vi "Main.vi"() -> ()   [LabVIEW 2013, in "Project Wizard.lvlib"]
doc: "This template is for the Queued Message Handler design pattern.\n\nThe Event Handling Loop generates messages based on user interface actions.\n\nThe Message Handling Loop processes messages generated by the Event Handling Loop, or by other messages. The messages are string values, so new messages can be added easily to the Message Cases case structure in the Message Handling Loop. Each message cluster can also provide an optional value for Message Data, which is a variant that can be converted to whatever message-specific data is required."
uses:
  Project Wizard.lvlib
  controls/UI Data.ctl
  controls/Template.ctl
  support/Message Queue/Enqueue Message (Single).vi
  support/Message Queue/Enqueue Message (Array).vi
  <vilib>/Platform/browser.llb/Open URL in Default Browser (path).vi
  <vilib>/Utility/error.llb/Error Cluster From Error Code.vi
  <vilib>/regexp/Match Regular Expression.xnode
  <vilib>/ErrorRing/Error Ring.xnode
  support/Message Queue/Message Queue.lvlib
  support/User Event - Stop/User Event - Stop.lvlib
panel:
  in  "Tab Control":enum32{"Project", "Properties"}(tab)
  in  "Target IP address or DNS name":string
  in  "Project name":string
  in  "Template":u16(ring) items=["Base", "Base - XNET"]
  in  "Project root folder":path
  in  "ProjFolder":bool
  out "Project path":path
  in  "OpenProj":bool
  in  "Description":string
  in  "Creator":string
  in  "Cancel":bool
  in  "Create":bool
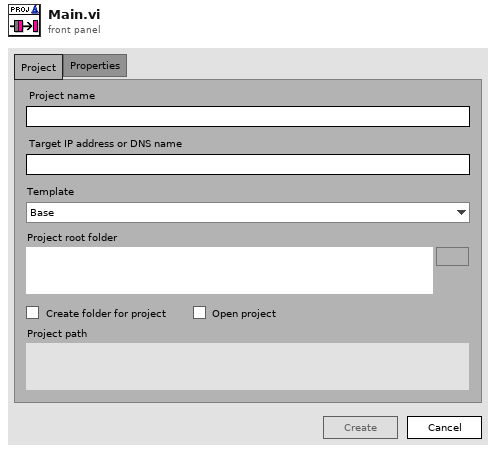
[diagram p1: front panel]
types:
  T1 = typedef "Project Wizard.lvlib/UI Data.ctl" = cluster{"ProjRootFolder":path, "ProjName":string, "Open":bool, "CreateFolder":bool, "Description":string, "Creator":string, "ProjPath":path, "Templates":T2[], "TemplateIdx":u16, "IP":string}
  T2 = typedef "Project Wizard.lvlib/Template.ctl" = cluster{"DispName":string, "Path":path, "DiskName":string}
  T3 = typedef "Project Wizard.lvlib/Message Queue.lvlib/All Message Queues.ctl" = cluster{"UI":refnum<queue>}
  T4 = enum8{"Enabled", "Disabled", "Disabled and Grayed Out"}
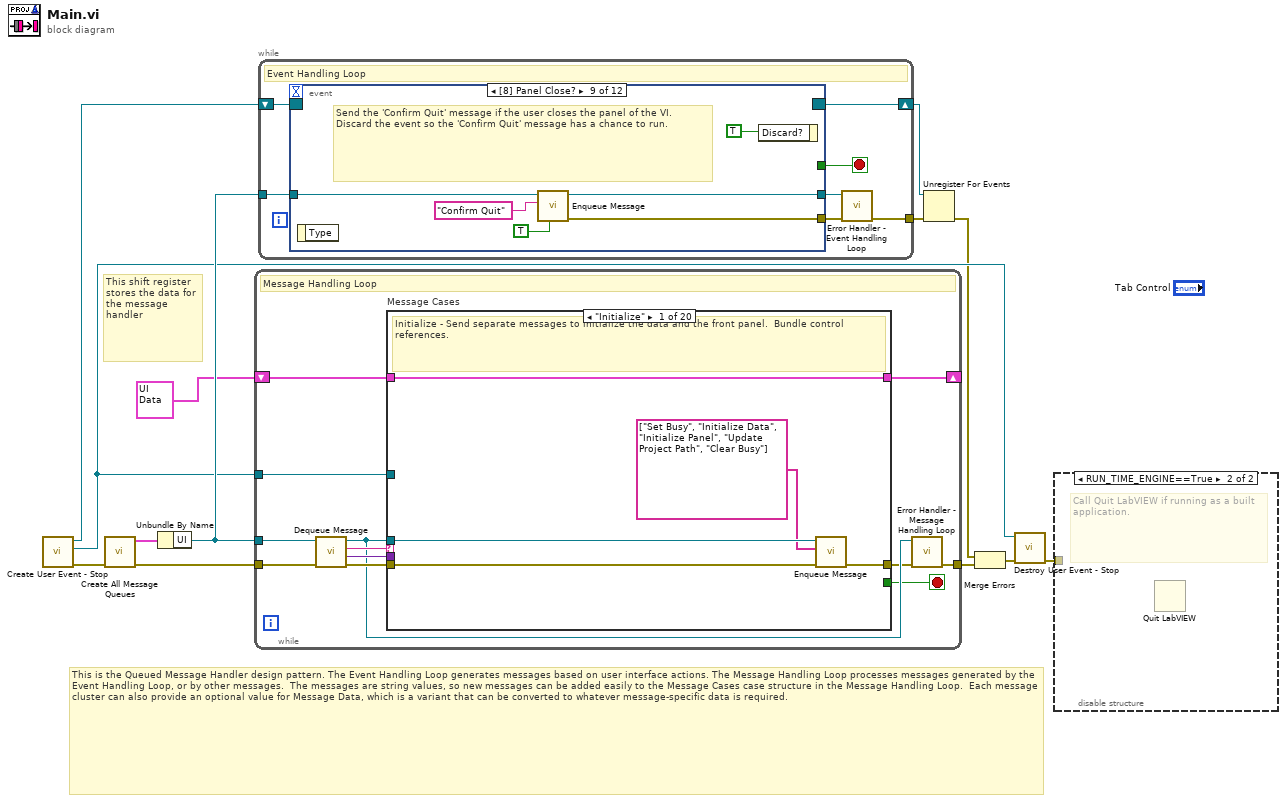
[diagram p0: block diagram]
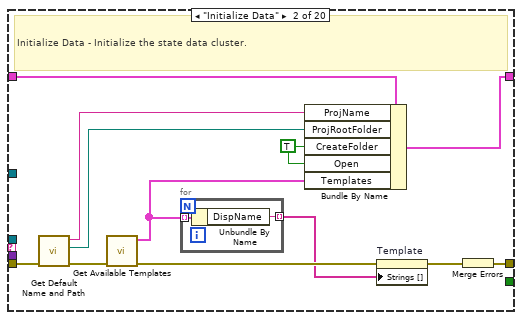
[diagram p2: hidden frame]
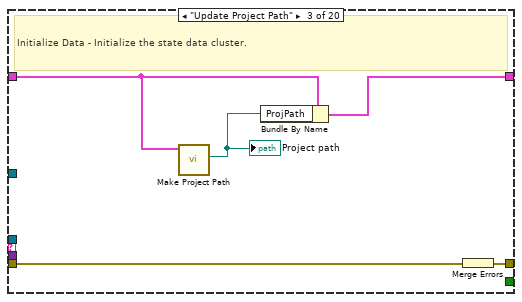
[diagram p3: hidden frame]
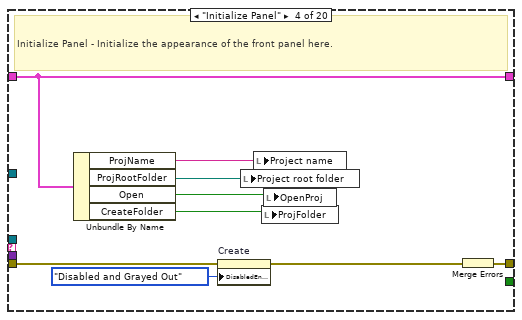
[diagram p4: hidden frame]
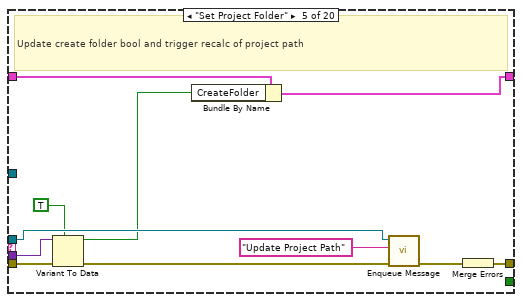
[diagram p5: hidden frame]
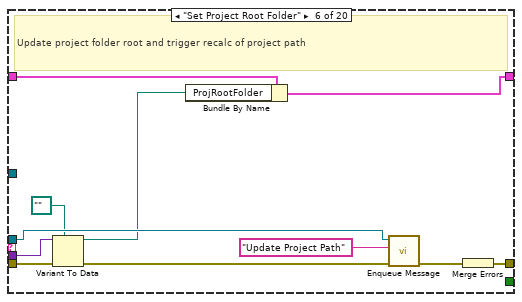
[diagram p6: hidden frame]
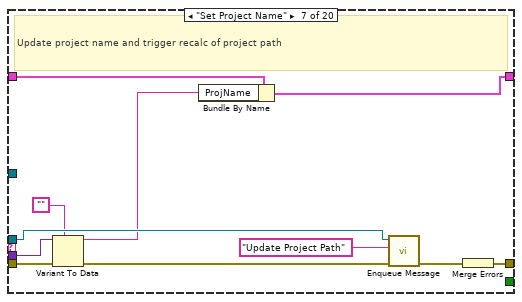
[diagram p7: hidden frame]
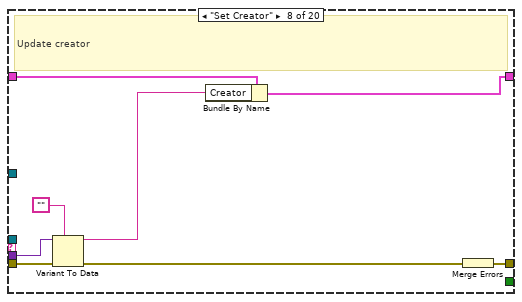
[diagram p8: hidden frame]
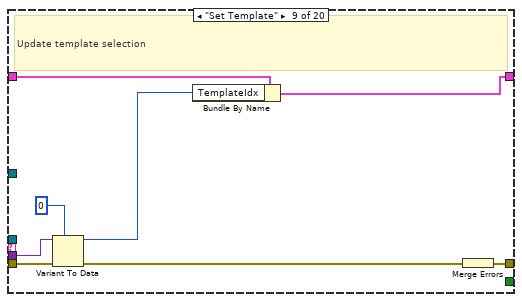
[diagram p9: hidden frame]
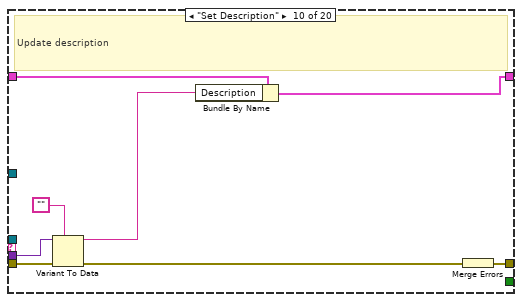
[diagram p10: hidden frame]
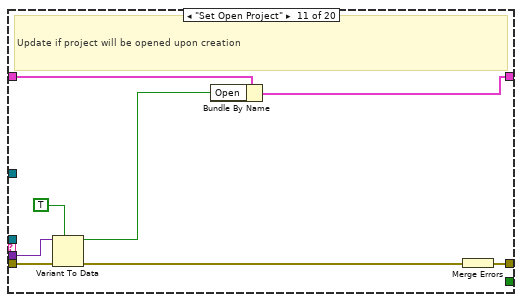
[diagram p11: hidden frame]
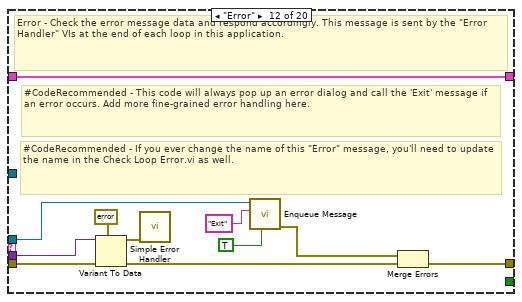
[diagram p12: hidden frame]
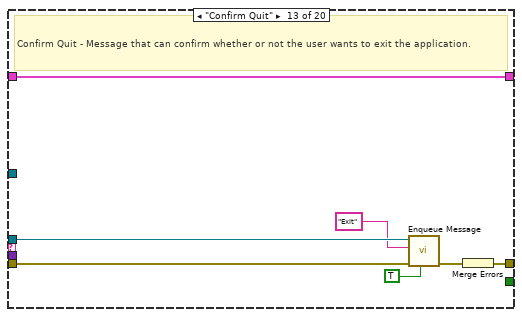
[diagram p13: hidden frame]
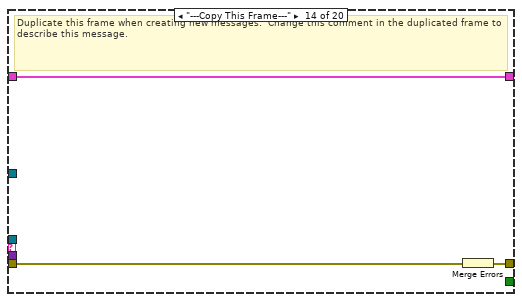
[diagram p14: hidden frame]
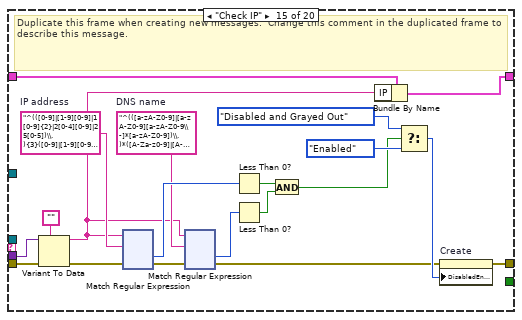
[diagram p15: hidden frame]
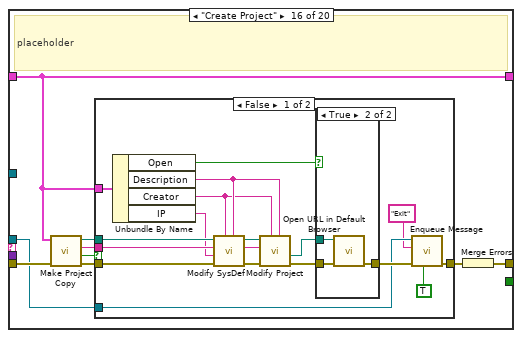
[diagram p16: hidden frame]
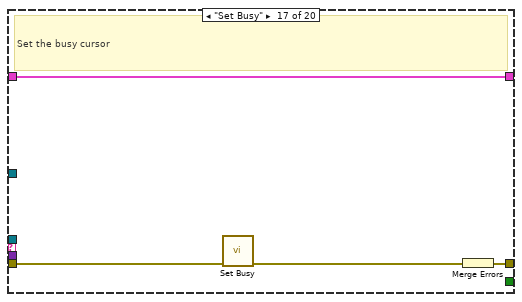
[diagram p19: hidden frame]
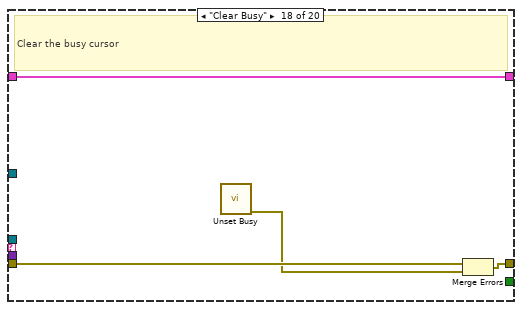
[diagram p20: hidden frame]
diagram:
  # "This shift register stores the data for the message handler"
  # "This is the Queued Message Handler design pattern. The Event Handling Loop generates messages based on user interface actions. The Message Handling Loop processes messages generated by the Event Handling Loop, or by other messages.  The messages are string values, so new messages can be added easily to the Message Cases case structure in the Message Handling Loop.  Each message cluster can also provide an optional value for Message Data, which is a variant that can be converted to whatever message-specific data is required."
  n1 = call "Create User Event - Stop.vi"() -> ("error out"=w7:errorcluster, "User Event - Stop"=w5:refnum<user-event>, "Stop Event Registration Refnum"=w8:refnum<event-registration>)  [unwired: 9 in]
  n2 = call "Create All Message Queues.vi"("error in (no error)"=w7) -> ("error out"=w12:errorcluster, "Message Queues out"=w11:T3)  [unwired: 9 in]
  n3 = Unbundle By Name(w11) -> ("UI"=w9:refnum<queue>)
  n4 = while {
    tunnel: w9 -> [w18]
    shift-right: [w24] -> _
    shift-left: T1 {"ProjRootFolder"=path "", "ProjName"="", "Open"=FALSE, "CreateFolder"=FALSE, "Description"="", "Creator"="", "ProjPath"=path "", "Templates"=[], "TemplateIdx"=0, "IP"=""} ("Data Cluster") -> [w25]
    tunnel: w5 -> [w23]
    tunnel: w12 -> [w22]
    tunnel: [w16] -> w10
    stop <- w14 stop-if-true
    # "Message Handling Loop"
    n5 = call "Dequeue Message.vi"("error in (no error)"=w22, "Message Queue"=w18) -> ("error out"=w21:errorcluster, "Message Data"=w19:variant, "Message"=w20:string, "dup Message Queue"=w17:refnum<queue>)  [unwired: 6 in]
    n6 = case "Message Cases" shown="\"Initialize\"" w20 {
      selector: w20 -> [_ _ _ _ _ _ _ _ _ _ _ _ _ _ _ _ _ _ _ w441]
      tunnel: w17 -> [w28 _ _ _ w65 w76 w87 _ _ _ _ w126 w137 _ _ w393 _ _ w440 _]
      tunnel: w21 -> [w29 w39 w48 w52 w67 w78 w89 w97 w105 w113 w121 w134 w141 w144 w159 w400 w428 w430 w435 _]
      tunnel: [w30 w40 w49 w57 w68 w79 w90 w98 w106 w114 w122 w127 w139 w142 w163 w401 w426 w431 w436 w442] -> w15
      tunnel: w25 -> [w26 w42 w47 w58 w69 w80 w91 w99 w107 w115 w123 w133 w140 w143 w164 w395 w427 w432 w439 w443]
      tunnel: [w26 w41 w46 w58 w60 w71 w82 w93 w101 w109 w117 w133 w140 w143 w146 w395 w427 w432 w439 w443] -> w24
      tunnel: [_ _ _ _ _ _ _ _ _ _ _ _ _ _ _ _ _ _ TRUE _] -> w14
      tunnel: w19 -> [_ _ _ _ w62 w73 w84 w95 w103 w111 w119 w132 _ _ w157 _ _ _ _ _]
      tunnel: w23 -> [_ _ _ _ _ _ _ _ _ _ _ _ _ _ _ _ _ _ w434 _]
      frame "Initialize" {
        # "Initialize - Send separate messages to initialize the data and the front panel.  Bundle control references."
        n7 = call-poly "Enqueue Message.vi"("error in (no error)"=w29, "Message Array"=string[] ["Set Busy", "Initialize Data", "Initialize Panel", "Update Project Path", "Clear Busy"], "Message Queue"=w28) -> ("error out"=w30:errorcluster)  [unwired: 7 in, 1 out]
      }
      frame "Initialize Data" {
        w36 = TRUE ("CreateFolder")
        # "Initialize Data - Initialize the state data cluster."
        n8 = call "Get Default Name and Path.vi"("error in (no error)"=w39) -> ("error out"=w35:errorcluster, "Project root folder"=w37:path, "Project name"=w38:string)  [unwired: 8 in]
        n9 = call "Get Available Templates.vi"("error in (no error)"=w35) -> ("error out"=w33:errorcluster, "Templates"=w32:T2[])  [unwired: 9 in]
        n10 = for {
          tunnel: w32 -> [w44] mode=indexing
          tunnel: [w43] -> w31 mode=indexing
          n11 = Unbundle By Name(w44) -> ("DispName"=w43:string)
        }
        n12 = Bundle By Name(cluster=w42, "ProjName"=w38, "ProjRootFolder"=w37, "CreateFolder"=w36, "Open"=w36, "Templates"=w32) -> (w41:T1)
        n13 = property on="Template" class="Ring (strict)"(error in=w33, "Strings []"=w31) -> (error out=w34:errorcluster)  [unwired: 1 in, 1 out]
        n14 = Merge Errors(w34) -> (w40:errorcluster)
      }
      frame "Update Project Path" {
        # "Initialize Data - Initialize the state data cluster."
        n15 = call "Make Project Path.vi"("Data Cluster"=w47) -> ("project path"=w45:path)  [unwired: 9 in, 1 out]
        "Project path" <- w45
        n16 = Bundle By Name(cluster=w47, "ProjPath"=w45) -> (w46:T1)
        n17 = Merge Errors(w48) -> (w49:errorcluster)
      }
      frame "Initialize Panel" {
        # "Initialize Panel - Initialize the appearance of the front panel here."
        n18 = Unbundle By Name(w58) -> ("ProjName"=w56:string, "ProjRootFolder"=w55:path, "Open"=w54:bool, "CreateFolder"=w53:bool)
        n19 = property on="Create" class="Bool"(error in=w52, "DisabledEnum"=T4."Disabled and Grayed Out" ("Disabled")) -> (error out=w50:errorcluster)  [unwired: 1 in, 1 out]
        n20 = local write "Project root folder"(w55) -> ()
        n21 = local write "Project name"(w56) -> ()
        n22 = local write "ProjFolder"(w53) -> ()
        n23 = local write "OpenProj"(w54) -> ()
        n24 = Merge Errors(w50) -> (w57:errorcluster)
      }
      frame "Set Project Folder" {
        # "Update create folder bool and trigger recalc of project path"
        n25 = Variant To Data(error in=w67, type=TRUE, Variant=w62) -> (data=w59:bool, error out=w63:errorcluster)
        n26 = Bundle By Name(cluster=w69, "CreateFolder"=w59) -> (w60:T1)
        n27 = call-poly "Enqueue Message.vi"("error in (no error)"=w63, "Message"="Update Project Path", "Message Queue"=w65) -> ("error out"=w66:errorcluster)  [unwired: 7 in, 1 out]
        n28 = Merge Errors(w66) -> (w68:errorcluster)
      }
      frame "Set Project Root Folder" {
        # "Update project folder root and trigger recalc of project path"
        n29 = Variant To Data(error in=w78, type=path "", Variant=w73) -> (data=w70:path, error out=w74:errorcluster)
        n30 = Bundle By Name(cluster=w80, "ProjRootFolder"=w70) -> (w71:T1)
        n31 = call-poly "Enqueue Message.vi"("error in (no error)"=w74, "Message"="Update Project Path", "Message Queue"=w76) -> ("error out"=w77:errorcluster)  [unwired: 7 in, 1 out]
        n32 = Merge Errors(w77) -> (w79:errorcluster)
      }
      frame "Set Project Name" {
        # "Update project name and trigger recalc of project path"
        n33 = Variant To Data(error in=w89, type="", Variant=w84) -> (data=w81:string, error out=w85:errorcluster)
        n34 = Bundle By Name(cluster=w91, "ProjName"=w81) -> (w82:T1)
        n35 = call-poly "Enqueue Message.vi"("error in (no error)"=w85, "Message"="Update Project Path", "Message Queue"=w87) -> ("error out"=w88:errorcluster)  [unwired: 7 in, 1 out]
        n36 = Merge Errors(w88) -> (w90:errorcluster)
      }
      frame "Set Creator" {
        # "Update creator"
        n37 = Variant To Data(error in=w97, type="", Variant=w95) -> (data=w92:string, error out=w96:errorcluster)
        n38 = Bundle By Name(cluster=w99, "Creator"=w92) -> (w93:T1)
        n39 = Merge Errors(w96) -> (w98:errorcluster)
      }
      frame "Set Template" {
        # "Update template selection"
        n40 = Variant To Data(error in=w105, type=u16 0, Variant=w103) -> (data=w100:u16, error out=w104:errorcluster)
        n41 = Bundle By Name(cluster=w107, "TemplateIdx"=w100) -> (w101:T1)
        n42 = Merge Errors(w104) -> (w106:errorcluster)
      }
      frame "Set Description" {
        # "Update description"
        n43 = Variant To Data(error in=w113, type="", Variant=w111) -> (data=w108:string, error out=w112:errorcluster)
        n44 = Bundle By Name(cluster=w115, "Description"=w108) -> (w109:T1)
        n45 = Merge Errors(w112) -> (w114:errorcluster)
      }
      frame "Set Open Project" {
        # "Update if project will be opened upon creation"
        n46 = Variant To Data(error in=w121, type=TRUE, Variant=w119) -> (data=w116:bool, error out=w120:errorcluster)
        n47 = Bundle By Name(cluster=w123, "Open"=w116) -> (w117:T1)
        n48 = Merge Errors(w120) -> (w122:errorcluster)
      }
      frame "Error" {
        # "#CodeRecommended - If you ever change the name of this \"Error\" message, you'll need to update the name in the Check Loop Error.vi as well."
        # "#CodeRecommended - This code will always pop up an error dialog and call the 'Exit' message if an error occurs. Add more fine-grained error handling here."
        # "Error - Check the error message data and respond accordingly. This message is sent by the \"Error Handler\" VIs at the end of each loop in this application."
        n49 = Variant To Data(error in=w134, type=errorcluster {"status"=FALSE, "code"=0, "source"=""} ("error constant"), Variant=w132) -> (data=w130:errorcluster, error out=w129:errorcluster)
        n50 = call <vilib>:"Simple Error Handler.vi"("error in (no error)"=w130) -> ()  [unwired: 4 in, 5 out]
        n51 = call-poly "Enqueue Message.vi"("Priority Message? (F)"=TRUE, "Message"="Exit", "Message Queue"=w126) -> ("error out"=w128:errorcluster)  [unwired: 7 in, 1 out]
        n52 = Merge Errors(w128, w129) -> (w127:errorcluster)
      }
      frame "Confirm Quit" {
        # "Confirm Quit - Message that can confirm whether or not the user wants to exit the application."
        n53 = call-poly "Enqueue Message.vi"("Priority Message? (F)"=TRUE, "error in (no error)"=w141, "Message"="Exit", "Message Queue"=w137) -> ("error out"=w138:errorcluster)  [unwired: 6 in, 1 out]
        n54 = Merge Errors(w138) -> (w139:errorcluster)
      }
      frame "---Copy This Frame---" {
        # "Duplicate this frame when creating new messages.  Change this comment in the duplicated frame to describe this message."
        n55 = Merge Errors(w144) -> (w142:errorcluster)
      }
      frame "Check IP" {
        w147 = "^(([a-zA-Z0-9]|[a-zA-Z0-9][a-zA-Z0-9\\-]*[a-zA-Z0-9])\\.)*([A-Za-z0-9]|[A-Za-z0-9][A-Za-z0-9\\-]*[A-Za-z0-9])$"  # DNS name
        w155 = "^(([0-9]|[1-9][0-9]|1[0-9]{2}|2[0-4][0-9]|25[0-5])\\.){3}([0-9]|[1-9][0-9]|1[0-9?]{2}|2[0-4][0-9]|25[0-5])$"  # IP address
        # "Duplicate this frame when creating new messages.  Change this comment in the duplicated frame to describe this message."
        n56 = Variant To Data(error in=w159, type="", Variant=w157) -> (data=w145:string, error out=w158:errorcluster)
        n57 = xnode "Match Regular Expression"("input string"=w145, "regular expression"=w155, "error in"=w158) -> ("offset past match"=w152:i32, "error out"=w154:errorcluster)  [unwired: 3 in, 3 out]
        n58 = xnode "Match Regular Expression"("input string"=w145, "regular expression"=w147, "error in"=w154) -> ("offset past match"=w151:i32, "error out"=w153:errorcluster)  [unwired: 3 in, 3 out]
        n59 = Less Than 0?(x=w152) -> (x < 0?=w150:bool)
        n60 = Less Than 0?(x=w151) -> (x < 0?=w149:bool)
        n61 = And(x=w150, y=w149) -> (x .and. y?=w148:bool)
        n62 = Bundle By Name(cluster=w164, "IP"=w145) -> (w146:T1)
        n63 = Select(t=T4."Disabled and Grayed Out" ("Disabled"), s=w148, f=T4."Enabled" ("Disabled")) -> (s? t:f=w160:T4)
        n64 = property on="Create" class="Bool"(error in=w153, "DisabledEnum"=w160) -> (error out=w163:errorcluster)  [unwired: 1 in, 1 out]
      }
      frame "Create Project" {
        # "placeholder"
        n65 = call "Make Project Copy.vi"("error in (no error)"=w400, "UI Data"=w395) -> ("error out"=w398:errorcluster, "Cancelled"=w399:bool, "Name out"=w396:string, "Project Root Path"=w397:path)  [unwired: 6 in]
        n66 = case shown="False" w399 {
          tunnel: w398 -> [w419 w424]
          tunnel: w397 -> [w418 _]
          tunnel: w396 -> [w417 _]
          tunnel: w395 -> [w413 _]
          tunnel: [w409 w424] -> w394
          tunnel: w393 -> [w407 _]
          frame False {
            n67 = Unbundle By Name(w413) -> ("Open"=w411:bool, "Description"=w404:string, "Creator"=w403:string, "IP"=w402:string)
            n68 = call "Modify SysDef.vi"("Description"=w404, "Creator"=w403, "error in (no error)"=w419, "IP"=w402, "Name"=w417, "Project Root Path"=w418) -> ("error out"=w416:errorcluster, "Name dup"=w415:string, "Project Root Path dup"=w414:path)  [unwired: 3 in]
            n69 = call "Modify Project.vi"("Description"=w404, "Creator"=w403, "error in (no error)"=w416, "Name"=w415, "Project Root Path"=w414) -> ("error out"=w412:errorcluster, "Project Path"=w405:path)  [unwired: 3 in, 2 out]
            n70 = case shown="True" w411 {
              tunnel: w412 -> [w420 w423]
              tunnel: w405 -> [_ w422]
              tunnel: [w420 w421] -> w410
              frame False {
              }
              frame True {
                n71 = call-poly <vilib>:"Open URL in Default Browser.vi"("error in (no error)"=w423, "path"=w422) -> ("error out"=w421:errorcluster)  [unwired: 4 in, 1 out]
              }
            }
            n72 = call-poly "Enqueue Message.vi"("Priority Message? (F)"=TRUE, "error in (no error)"=w410, "Message"="Exit", "Message Queue"=w407) -> ("error out"=w409:errorcluster)  [unwired: 6 in, 1 out]
          }
          frame True {
          }
        }
        n73 = Merge Errors(w394) -> (w401:errorcluster)
      }
      frame "Set Busy" {
        # "Set the busy cursor"
        n74 = call <vilib>:"Set Busy.vi"("error in (no error)"=w428) -> ("error out"=w425:errorcluster)  [unwired: 9 in, 1 out]
        n75 = Merge Errors(w425) -> (w426:errorcluster)
      }
      frame "Clear Busy" {
        # "Clear the busy cursor"
        n76 = call <vilib>:"Unset Busy.vi"() -> ("error out"=w429:errorcluster)  [unwired: 11 in]
        n77 = Merge Errors(w430, w429) -> (w431:errorcluster)
      }
      frame "Exit" {
        # "Stop the VI"
        # "Release the message queue reference"
        # "Exit - Exit the application."
        n78 = call "Fire User Event - Stop.vi"("User Event - Stop"=w434) -> ("error out"=w433:errorcluster)  [unwired: 10 in]
        n79 = Release Queue(queue=w440, error in (no error)=w435) -> (error out=w437:errorcluster)  [unwired: 1 in, 2 out]
        n80 = Merge Errors(w433, w437) -> (w436:errorcluster)
      }
      frame Default {
        # "'Default' case only runs if there is a message that isn't defined in any of the other cases.  Output a programming error."
        n81 = xnode "Error Ring"("parameter 0"=w441) -> ("error out"=w442:errorcluster)
      }
    }
    n82 = call "Error Handler - Message Handling Loop.vi"("error in (no error)"=w15, "Message Queue"=w17) -> ("dup error in"=w16:errorcluster)  [unwired: 8 in, 1 out]
  }
  n83 = while {
    tunnel: w9 -> [w457]
    shift-right: [w455] -> w3
    shift-left: w8 -> [w456]
    tunnel: [w451] -> w1
    stop <- w453 stop-if-true
    # "Event Handling Loop"
    n84 = event shown="[8] Panel Close?" {
      selector: w456 -> [_ _ _ _ _ _ _ _ _ _ _ _]
      dyn-events: [_ _ _ _ _ _ _ _ _ _ _ _] -> w455
      timeout: _ -> [_ _ _ _ _ _ _ _ _ _ _ _]
      tunnel: [_ _ _ _ _ _ _ _ _ _ _ TRUE ("Discard?")] -> w453
      tunnel: w457 -> [w462 w467 w472 w477 w482 w487 w492 w497 w502 w508 w512 w514]
      tunnel: [w459 w464 w469 w474 w479 w484 w489 w494 w501 w507 w511 _] -> w454
      tunnel: [w461 w466 w471 w476 w481 w486 w491 w496 w500 w506 w510 w514] -> w452
      event "ProjFolder": Value Change {
        n85 = event-data() -> ("NewVal"=w458:bool)  [unwired: 1 in]
        n86 = call-poly "Enqueue Message.vi"("Message Data"=w458, "Message"="Set Project Folder", "Message Queue"=w462) -> ("error out"=w459:errorcluster, "dup Message Queue"=w461:refnum<queue>)  [unwired: 7 in]
      }
      event "Project root folder": Value Change {
        n87 = event-data() -> ("NewVal"=w463:path)  [unwired: 1 in]
        n88 = call-poly "Enqueue Message.vi"("Message Data"=w463, "Message"="Set Project Root Folder", "Message Queue"=w467) -> ("error out"=w464:errorcluster, "dup Message Queue"=w466:refnum<queue>)  [unwired: 7 in]
      }
      event "Project name": Value Change {
        n89 = event-data() -> ("NewVal"=w468:string)  [unwired: 1 in]
        n90 = call-poly "Enqueue Message.vi"("Message Data"=w468, "Message"="Set Project Name", "Message Queue"=w472) -> ("error out"=w469:errorcluster, "dup Message Queue"=w471:refnum<queue>)  [unwired: 7 in]
      }
      event "Target IP address or DNS name": Value Change {
        n91 = event-data() -> ("NewVal"=w473:string)  [unwired: 1 in]
        n92 = call-poly "Enqueue Message.vi"("Message Data"=w473, "Message"="Check IP", "Message Queue"=w477) -> ("error out"=w474:errorcluster, "dup Message Queue"=w476:refnum<queue>)  [unwired: 7 in]
      }
      event "Template": Value Change {
        n93 = event-data() -> ("NewVal"=w478:u16)  [unwired: 1 in]
        n94 = call-poly "Enqueue Message.vi"("Message Data"=w478, "Message"="Set Template", "Message Queue"=w482) -> ("error out"=w479:errorcluster, "dup Message Queue"=w481:refnum<queue>)  [unwired: 7 in]
      }
      event "Creator": Value Change {
        n95 = event-data() -> ("NewVal"=w483:string)  [unwired: 1 in]
        n96 = call-poly "Enqueue Message.vi"("Message Data"=w483, "Message"="Set Creator", "Message Queue"=w487) -> ("error out"=w484:errorcluster, "dup Message Queue"=w486:refnum<queue>)  [unwired: 7 in]
      }
      event "Description": Value Change {
        n97 = event-data() -> ("NewVal"=w488:string)  [unwired: 1 in]
        n98 = call-poly "Enqueue Message.vi"("Message Data"=w488, "Message"="Set Description", "Message Queue"=w492) -> ("error out"=w489:errorcluster, "dup Message Queue"=w491:refnum<queue>)  [unwired: 7 in]
      }
      event "OpenProj": Value Change {
        n99 = event-data() -> ("NewVal"=w493:bool)  [unwired: 1 in]
        n100 = call-poly "Enqueue Message.vi"("Message Data"=w493, "Message"="Set Open Project", "Message Queue"=w497) -> ("error out"=w494:errorcluster, "dup Message Queue"=w496:refnum<queue>)  [unwired: 7 in]
      }
      event Panel Close? {
        # "Send the 'Confirm Quit' message if the user closes the panel of the VI. Discard the event so the 'Confirm Quit' message has a chance to run."
        n101 = event-data() -> ()  [unwired: 1 in, 1 out]
        n102 = call-poly "Enqueue Message.vi"("Priority Message? (F)"=TRUE, "Message"="Confirm Quit", "Message Queue"=w502) -> ("error out"=w501:errorcluster, "dup Message Queue"=w500:refnum<queue>)  [unwired: 7 in]
        n103 = event-data("Discard?"=TRUE) -> ()  [unwired: 1 in, 1 out]
      }
      event "Cancel": Value Change {
        n104 = event-data() -> ()  [unwired: 1 in, 1 out]
        n105 = call-poly "Enqueue Message.vi"("Priority Message? (F)"=TRUE, "Message"="Exit", "Message Queue"=w508) -> ("error out"=w507:errorcluster, "dup Message Queue"=w506:refnum<queue>)  [unwired: 7 in]
      }
      event "Create": Value Change {
        n106 = event-data() -> ()  [unwired: 1 in, 1 out]
        n107 = call-poly "Enqueue Message.vi"("Message Array"=string[] ["Set Busy", "Create Project", "Clear Busy"], "Message Queue"=w512) -> ("error out"=w511:errorcluster, "dup Message Queue"=w510:refnum<queue>)  [unwired: 8 in]
      }
      event User Event {
        # "The Message Handling Loop processed an \"Exit\" message, which fired this event to stop the Event Handling Loop."
        n108 = event-data() -> ()  [unwired: 1 in, 1 out]
      }
    }
    n109 = call "Error Handler - Event Handling Loop.vi"("error in (no error)"=w454, "Message Queue"=w452) -> ("dup error in"=w451:errorcluster)  [unwired: 8 in, 1 out]
  }
  n110 = Unregister For Events(event registration refnum=w3, error in=w1) -> (error out=w4:errorcluster)
  n111 = Merge Errors(w4, w10) -> (w6:errorcluster)
  n112 = call "Destroy User Event - Stop.vi"("error in (no error)"=w6, "User Event - Stop"=w5) -> ("error out"=w13:errorcluster)  [unwired: 9 in]
  n113 = disable-structure shown="RUN_TIME_ENGINE==True" {
    disable-tunnel: w13 -> [_ _]
    frame condition #0 (active) {
    }
    frame condition #1 {
      # "Call Quit LabVIEW if running as a built application."
      n114 = Quit LabVIEW() -> ()  [unwired: 1 in]
    }
  }
